vi "FindImplementation.vi"(3 "error in (no error)":errorcluster, 4 "Method Name":string, 5 "Class Refnum":refnum<vi>) -> (0 "error out":errorcluster, 1 "VI Reference":refnum<vi>, 2 "Class out":refnum<vi>)   [LabVIEW 2017, in "DynamicDispatchImplementationWalker.lvlib"]
uses:
  DynamicDispatchImplementationWalker.lvlib
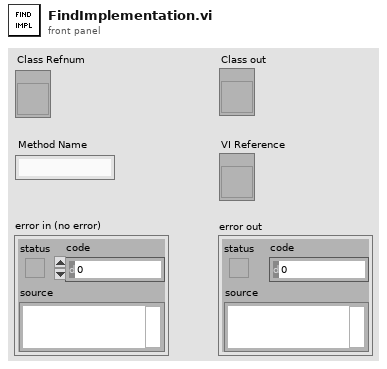
[diagram p1: front panel]
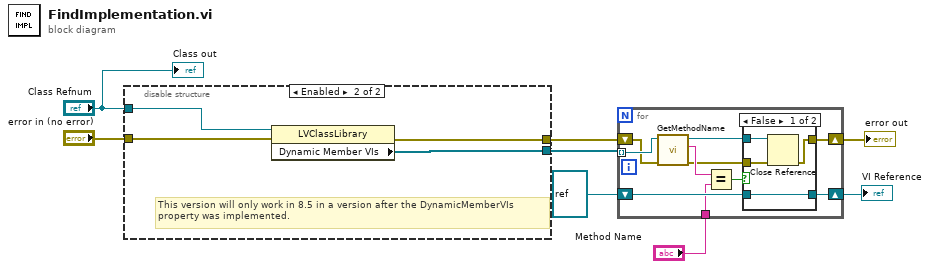
[diagram p0: block diagram]
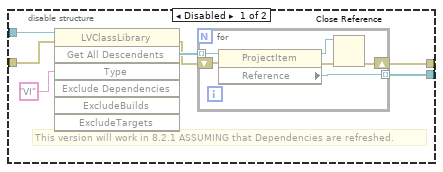
[diagram p2: hidden frame]
diagram:
  n1 = disable-structure shown="Enabled" {
    disable-tunnel: "error in (no error)" -> [w15 w24]
    disable-tunnel: "Class Refnum" -> [w13 w25]
    disable-tunnel: [w11 w23] -> w2
    disable-tunnel: [w9 w22] -> w1
    frame Disabled {
      # "This version will work in 8.2.1 ASSUMING that Dependencies are refreshed."
      n2 = invoke class="LVClassLibrary" method="Get All Descendents"(reference=w13, error in=w15, "Type"="VI") -> (error out=w10:errorcluster, "All Descendents"=w12:refnum<vi>[])  [unwired: 4 in, 5 out]
      n3 = for {
        tunnel: w12 -> [w21] mode=indexing
        tunnel: [w20] -> w11 mode=indexing
        shift-right: [w18] -> w9
        shift-left: w10 -> [w19]
        n4 = property class="ProjectItem"(reference=w21, error in=w19) -> (reference out=w16:refnum<vi>, error out=w17:errorcluster, "Reference"=w20:refnum<vi>)
        n5 = Close Reference(reference=w16, error in (no error)=w17) -> (error out=w18:errorcluster)
      }
    }
    frame Enabled {
      # "This version will only work in 8.5 in a version after the DynamicMemberVIs\nproperty was implemented."
      n6 = property class="LVClassLibrary"(reference=w25, error in=w24) -> (error out=w22:errorcluster, "Dynamic Member VIs"=w23:refnum<vi>[])  [unwired: 1 out]
    }
  }
  n7 = for {
    shift-right: [w31] -> w6
    shift-left: w1 -> [w27]
    shift-right: [w34] -> w8
    shift-left: refnum<vi> refnum ("Reference") -> [w33]
    tunnel: "Method Name" -> [w32]
    tunnel: w2 -> [w30] mode=indexing
    n8 = call "GetMethodName.vi"("error in (no error)"=w27, "VI Reference"=w30) -> ("error out"=w26:errorcluster, "Method Name"=w28:string, "VI Reference out"=w29:refnum<vi>)  [unwired: 7 in]
    n9 = Equal?(x=w28, y=w32) -> (x = y?=w35:bool)
    n10 = case shown="False" w35 {
      tunnel: w26 -> [w39 w41]
      tunnel: w29 -> [w38 w40]
      tunnel: [w37 w41] -> w31
      tunnel: [w36 w40] -> w34
      tunnel: w33 -> [w36 _]
      frame False {
        n11 = Close Reference(reference=w38, error in (no error)=w39) -> (error out=w37:errorcluster)
      }
      frame True {
      }
    }
  }
  "VI Reference" <- w8
  "error out" <- w6
  "Class out" <- "Class Refnum"
